vi "Disconnect.vi"(7 "path in":path, 8 "error in (no error)":errorcluster, 10 "addr_":string, 11 "s_":u64) -> (0 "error out":errorcluster, 3 "s_ out":u64)   [LabVIEW 2025, in "LibZMQ.lvlib"]
doc: "ZMQ_EXPORT int zmq_disconnect (void *s_, const char *addr_);\n\nDisconnect from an endpoint"
uses:
  LibZMQ.lvlib
  errno.vi
  strerror.vi
  <vilib>/Utility/error.llb/Error Cluster From Error Code.vi
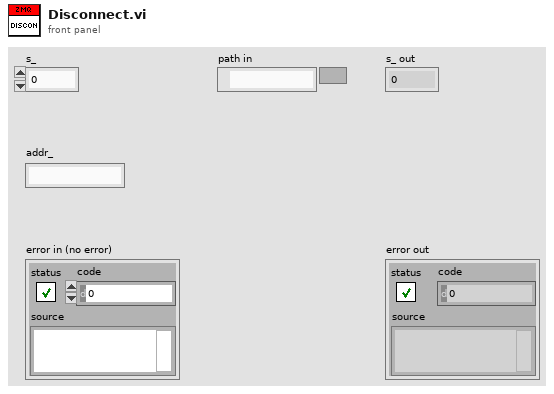
[diagram p1: front panel]
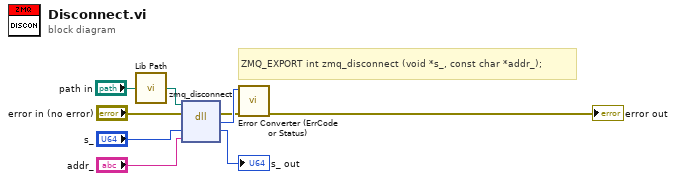
[diagram p0: block diagram]
diagram:
  # "ZMQ_EXPORT int zmq_disconnect (void *s_, const char *addr_);"
  n1 = call "Lib Path.vi"("path override"="path in") -> ("lib path"=w1:path)
  n2 = dll-call lib="libzmq-v143-mt-4_3_6.*" fn="zmq_disconnect"(path in=w1, error in="error in (no error)", "s_"="s_", "addr_"="addr_") -> (error out=w4:errorcluster, "return type"=w9:i32, "s_"=→"s_ out":u64)  [unwired: 2 in, 1 out]
  n3 = call "Error Converter (ErrCode or Status).vi"("error in (no error)"=w4, "error code"=w9) -> ("error out"=→"error out":errorcluster)  [unwired: 9 in]
